vi "SOFT.vi"() -> ()   [LabVIEW 2020]
uses:
  <vilib>/regexp/Match Regular Expression.xnode
panel:
  in  "Combo Box":string(combo)
  in  "branche":i32
  out "APPL":string
  out "ESW":string
  out "CONFIG":string
  out "ASW":string
  out "folder names":string[](array[string])
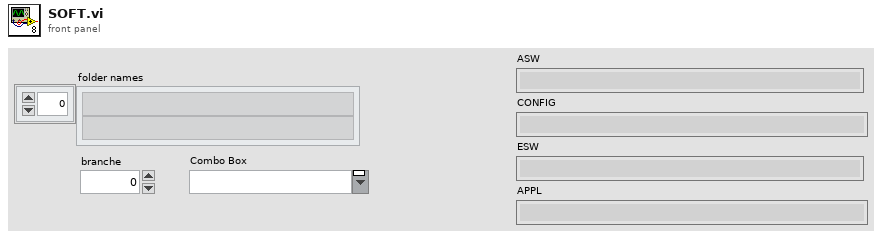
[diagram p1: front panel]
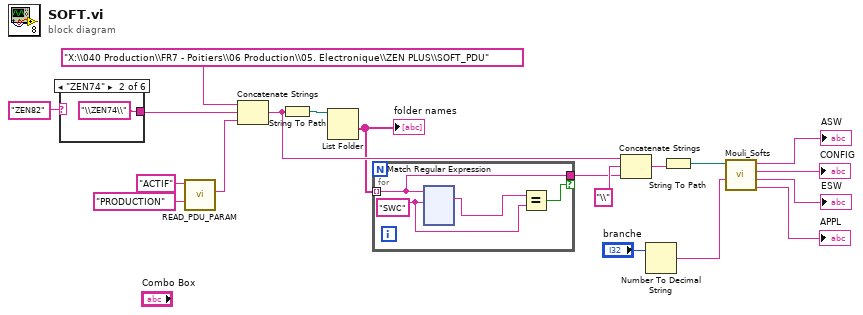
[diagram p0: block diagram]
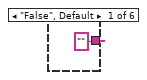
[diagram p2: hidden frame]
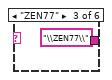
[diagram p3: hidden frame]
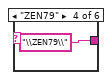
[diagram p4: hidden frame]
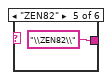
[diagram p5: hidden frame]
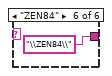
[diagram p6: hidden frame]
diagram:
  n1 = case shown="\"ZEN74\"" "ZEN82" {
    tunnel: ["" "\\ZEN74\\" "\\ZEN77\\" "\\ZEN79\\" "\\ZEN82\\" "\\ZEN84\\"] -> w17
    frame "False", Default {
    }
    frame "ZEN74" {
    }
    frame "ZEN77" {
    }
    frame "ZEN79" {
    }
    frame "ZEN82" {
    }
    frame "ZEN84" {
    }
  }
  n2 = call <userlib>:"READ_PDU_PARAM.vi"("section"="PRODUCTION", "key"="ACTIF") -> ("str"=w14:string)  [unwired: 5 in, 4 out]
  n3 = Concatenate Strings("X:\\040 Production\\FR7 - Poitiers\\06 Production\\05. Electronique\\ZEN PLUS\\SOFT_PDU", w17, w14) -> (w12:string)
  n4 = String To Path(string=w12) -> (path=w13:path)
  n5 = List Folder(path=w13) -> (folder names=w4:string[])  [unwired: 3 in, 3 out]
  "folder names" <- w4
  n6 = for {
    tunnel: w4 -> [w29] mode=indexing
    tunnel: [w29] -> w3 if=w28
    w27 = "SWC" ("regular expression")
    n7 = xnode "Match Regular Expression"("input string"=w29, "regular expression"=w27) -> ("whole match"=w26:string)  [unwired: 4 in, 4 out]
    n8 = Equal?(x=w26, y=w27) -> (x = y?=w28:bool)
  }
  n9 = Concatenate Strings(w12, "\\" ("string"), w3) -> (w11:string)
  n10 = Number To Decimal String(number="branche") -> (decimal integer string=w2:string)  [unwired: 1 in]
  n11 = String To Path(string=w11) -> (path=w10:path)
  n12 = call "Mouli_Softs.vi"("Branche"=w2, "chemin"=w10) -> ("APPL"=→"APPL":string, "ESW"=→"ESW":string, "CONFIG"=→"CONFIG":string, "ASW"=→"ASW":string)  [unwired: 6 in]
